vi "Configure OVP.vi"(8 "error in (no error)":errorcluster, 10 "Overvoltage Protection Value (110.0 V)":dbl=110.0 format="%_4g", 11 "VISA resource name":refnum<visa-resource-name>) -> (0 "error out":errorcluster, 3 "VISA resource name out":refnum<visa-resource-name>)   [LabVIEW 2020]
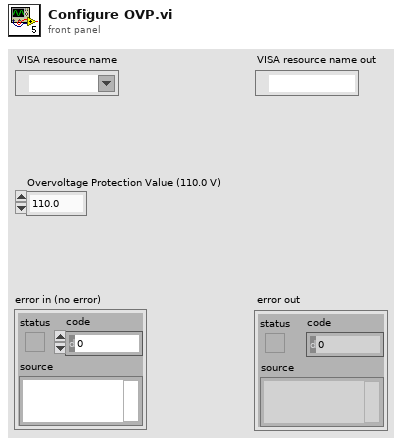
[diagram p1: front panel]
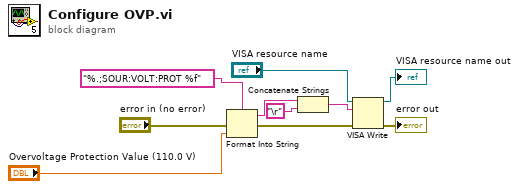
[diagram p0: block diagram]
diagram:
  n1 = Format Into String(format string="%.;SOUR:VOLT:PROT %f", error in="error in (no error)", "Overvoltage Protection Value (110.0 V)") -> (resulting string=w1:string, error out=w7:errorcluster)  [unwired: 1 in]
  n2 = Concatenate Strings(w1, "\r") -> (w4:string)
  n3 = VISA Write(VISA resource name="VISA resource name", write buffer=w4, error in (no error)=w7) -> (VISA resource name out=→"VISA resource name out":refnum<visa-resource-name>, error out=→"error out":errorcluster)  [unwired: 1 out]
